vi "CreateSubVIPackage.vi"(4 "SubVIs path":path, 5 "SubVIs":variant, 6 "error in":errorcluster) -> (0 "error out":errorcluster)   [LabVIEW 2014, in "PyConvBD.lvclass"]
uses:
  PyConvBD.lvclass
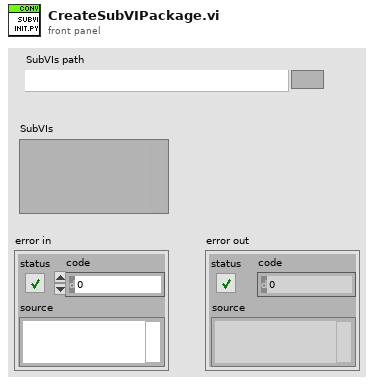
[diagram p1: front panel]
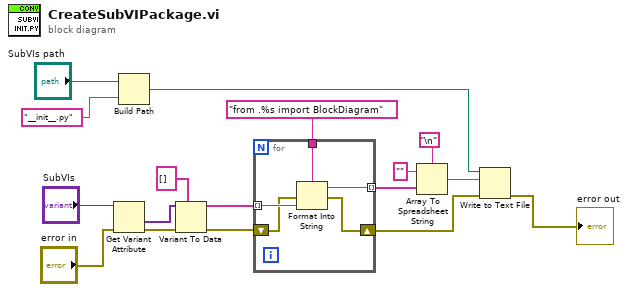
[diagram p0: block diagram]
diagram:
  n1 = Get Variant Attribute(Variant="SubVIs", error in="error in") -> (values=w15:variant[], error out=w16:errorcluster)  [unwired: 2 in, 2 out]
  n2 = Build Path(base path="SubVIs path", name or relative path="__init__.py") -> (appended path=w2:path)
  n3 = Variant To Data(error in=w16, type=string[] [], Variant=w15) -> (data=w13:string[], error out=w11:errorcluster)
  n4 = for {
    tunnel: w13 -> [w22] mode=indexing
    shift-right: [w21] -> w3
    shift-left: w11 -> [w20]
    tunnel: "from .%s import BlockDiagram" ("format string") -> [w19]
    tunnel: [w18] -> w9 mode=indexing
    n5 = Format Into String(format string=w19, error in=w20, w22) -> (resulting string=w18:string, error out=w21:errorcluster)  [unwired: 1 in]
  }
  n6 = Array To Spreadsheet String(delimiter (Tab)="\n", array=w9, 3:"" ("format string")) -> (spreadsheet string=w4:string)
  n7 = Write to Text File(file (use dialog)=w2, text=w4, error in=w3) -> (error out=→"error out":errorcluster)  [unwired: 1 in, 2 out]
